vi "Destroy.vi"(0 "reference in":refnum<class "DemoSubClass2.lvclass">, 5 "error in (no error)":errorcluster) -> (14 "reference out":refnum<class "DemoSubClass2.lvclass">, 19 "error out":errorcluster)   [LabVIEW 2020, in "DemoSubClass2.lvclass"]
uses:
  DemoSubClass2.lvclass
  C:/Program Files (x86)/National Instruments/LabVIEW 2020/vi.lib/addons/_AddQ/G#Object/G#Object.lvclass
  DemoClass1_class/DemoClass1.lvclass
  <vilib>/addons/_AddQ/G#Object/G#Object.lvclass
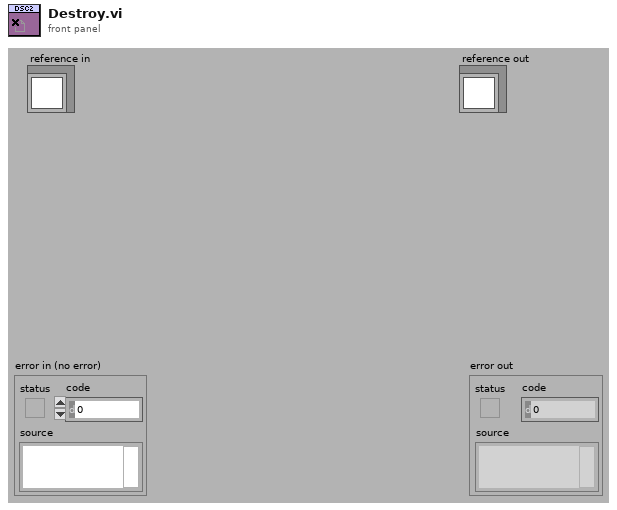
[diagram p1: front panel]
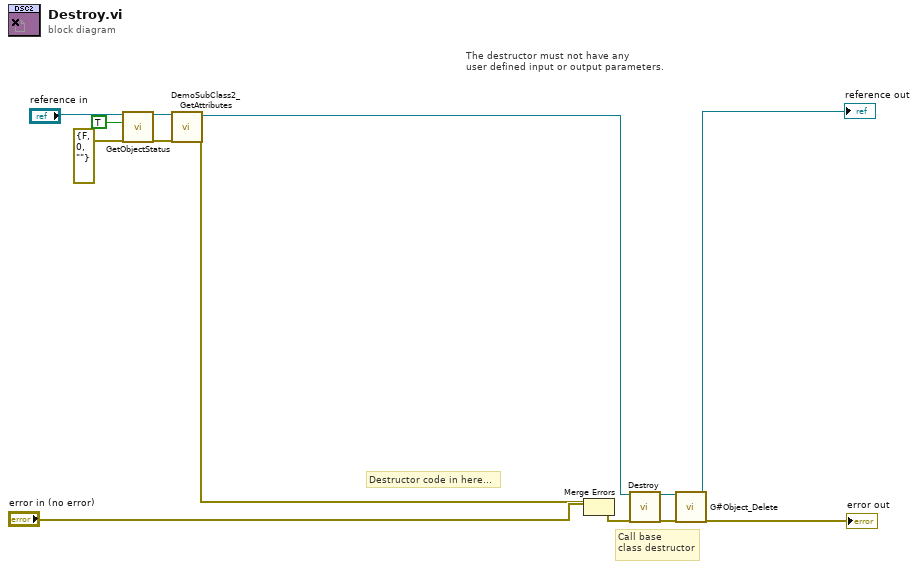
[diagram p0: block diagram]
diagram:
  # "Destructor code in here..."
  # "The destructor must not have any\nuser defined input or output parameters."
  # "Call base\nclass destructor"
  n1 = call-dynamic "GetObjectStatus.vi"("reference in"="reference in", "simple info (F)"=TRUE ("Simple Info"), "error in (no error)"=errorcluster {"status"=FALSE, "code"=0, "source"=""}) -> ("reference out"=w5:refnum<class "DemoSubClass2.lvclass">, "error out"=w3:errorcluster)  [unwired: 5 in, 10 out]
  n2 = call "DemoSubClass2_GetAttributes.vi"("reference in"=w5, "error in (no error)"=w3) -> ("reference out"=w9:refnum<class "DemoSubClass2.lvclass">, "error out"=w6:errorcluster)  [unwired: 1 in, 15 out]
  n3 = Merge Errors("error in (no error)", w6) -> (w12:errorcluster)
  n4 = call-parent "Destroy.vi"("reference in"=w9, "error in (no error)"=w12) -> ("reference out"=w8:refnum<class "DemoSubClass2.lvclass">, "error out"=w11:errorcluster)  [unwired: 16 out]
  n5 = call <vilib>:"G#Object_Delete.vi"("reference in"=w8, "error in (no error)"=w11) -> ("reference out"=→"reference out":refnum<class "DemoSubClass2.lvclass">, "error out"=→"error out":errorcluster)  [unwired: 16 in]
